vi "Roller Button Read.vi"(7 "Driver Button Cluster":T1, 9 "D-Pad":T2, 10 "Button Cluster":T1, 11 "Axes":T3) -> ()   [LabVIEW 2015]
uses:
  Real-Life Controls/Axes Cluster.ctl
  Real-Life Controls/D-Pad.ctl
  Real-Life Controls/Button Cluster.ctl
  Roller Modes.ctl
  Common Code/Auto Roller Commands.ctl
  Common Code/Roller Mode Enum.ctl
  Really Real Manual Align.ctl
  Common Code/Elevator State.ctl
  Common Code/Change Detect.vi
  Common Code/Change Detect Boolean.vi
  Robot Global Data.vi
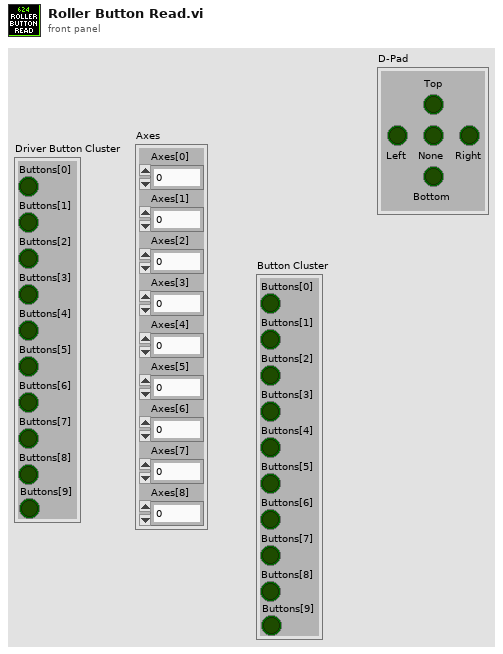
[diagram p1: front panel]
types:
  T1 = typedef "Button Cluster.ctl" = cluster{"Buttons[0]":bool, "Buttons[1]":bool, "Buttons[2]":bool, "Buttons[3]":bool, "Buttons[4]":bool, "Buttons[5]":bool, "Buttons[6]":bool, "Buttons[7]":bool, "Buttons[8]":bool, "Buttons[9]":bool}
  T2 = typedef "D-Pad.ctl" = cluster{"Top":bool, "Bottom":bool, "None":bool, "Right":bool, "Left":bool}
  T3 = typedef "Axes Cluster.ctl" = cluster{"Axes[0]":dbl, "Axes[1]":dbl, "Axes[2]":dbl, "Axes[3]":dbl, "Axes[4]":dbl, "Axes[5]":dbl, "Axes[6]":dbl, "Axes[7]":dbl, "Axes[8]":dbl}
  T4 = typedef "Elevator State.ctl" = enum16{"Idle", "Goto Load Position", "Wait for Load", "Load Drop", "Load Lift", "Drop Stack", "Goto Eject Position", "Eject ", "Raise Trashcan", "Open Stabilizer", "Untip Drop", "Untip Wait", "Untip Lift", "Abort Load", "HP Load Wait", "HP Load Drop", "HP Load Lift", "HP Load Abort", "Close Stabilizer", "HP Load Unfinish", "HP Load Score", "HP Load Finish", "HP Goto Finish Down", "HP Goto Finish Up", "Full"}
  T5 = typedef "Really Real Manual Align.ctl" = enum16{"In", "Left", "Right", "Out", "Idle", "HP Load", "Speeds"}
  T6 = typedef "Auto Roller Commands.ctl" = enum16{"Drag Tote", "Grab Tote", "Idle", "Eject Tote", "Untip Can", "Grab Can"}
  T7 = typedef "Roller Modes.ctl" = cluster{"Auto Roller Command":T6, "Roller Mode":T8, "Override Intake Speed":dbl}
  T8 = typedef "Roller Mode Enum.ctl" = enum16{"Manual", "Safe", "Auto"}
  T9 = typedef "Elevator Status.ctl" = cluster{"Height":dbl, "Enc Value":dbl, "Limit Override":bool, "Mode":T10, "High IR":bool, "Motor Out":dbl, "Ping Detect":bool, "Auto Elevator Indicators":T11, "Master Current":dbl, "Slave Current":dbl, "High Current":bool, "Current Tripped":bool, "Top Limit":bool, "Bottom Limit":bool, "Eject Piston":bool, "Stabilizer":bool, "Finger":bool, "Finger Height":dbl, "Finger Raw":dbl, "Finger at Bottom":bool}
  T10 = typedef "Elevator Mode.ctl" = enum16{"Manual", "Safe", "Auto"}
  T11 = typedef "Auto Elevator Indicators.ctl" = cluster{"Target Out":dbl, "Storing Trashcan?":bool, "State":T4, "In Range":bool, "Store Can Command":bool, "HP Load":bool}
  T12 = typedef "Dashboard Control Data.ctl" = cluster{"Cam Exposure":dbl, "Go to angle":dbl, "Steer PID Gains":cluster{"proportional gain (Kc)":dbl, "integral time (Ti, min)":dbl, "derivative time (Td, min)":dbl}, "Steer PID output Range":cluster{"output high":dbl, "output low":dbl}, "Pressure m \nValue":dbl, "Pressure b \nValue":dbl, "Roller Command Cluster ":T13, "Elevator":T14, "Encoder Control":T16, "Auton Settings":cluster{"Drive Dist Window Size":dbl}, "Drivetrain Settings":T17, "Lance":T18}
  T13 = typedef "Roller Control.ctl" = cluster{"Intake Speed":dbl, "Turn In Speed":dbl, "Unload Speed":dbl, "Turn Out Speed":dbl, "Ping Align Tolerance":dbl, "Tote Range Threshold":dbl, "Right Pot 0":dbl, "Pot Threshold":dbl, "Left Pot 0":dbl, "Right Pot Scale":dbl, "Left Pot Scale":dbl, "Min Elevator Height":dbl, "Eject Time":dbl, "Eject US Threshold":dbl, "Anti-Twitch Time":u32, "Ping Caring Threshold":dbl, "Pot Diff Threshold":dbl, "Pinch Sustain":u32, "Absorb Give Up Threshold":dbl, "Untip In Threshold":dbl, "Untip Grab Range":dbl, "Ultrasonic Hold Time":u32, "Landscape Absorb Time":u32, "Pot Use Wait Time":u32, "Can Turn Stop Range":dbl, "HP Load Speed":dbl, "Stick Multiplier":dbl, "Coop Eject Speed":dbl}
  T14 = typedef "Elevator DB Control.ctl" = cluster{"PID Output Range":cluster{"output high":dbl, "output low":dbl}, "PID gains":cluster{"proportional gain (Kc)":dbl, "integral time (Ti, min)":dbl, "derivative time (Td, min)":dbl}, "Height Tolerance":sgl, " Encoder Constant":dbl, "Eject Time":sgl, "Zeroing Speed":sgl, "Presets":T15, "Ping Detect Threshold":sgl, "Trashcan Detect Threshold":sgl, "Zero Filter Time":dbl, "Stabilizer Open Time":dbl, "Zero Creep Speed":dbl, "Max Current":dbl, "Current Trip Time":dbl, "Abort Pitch":dbl, "Finger m":dbl, "Finger b":dbl, "Finger max ":dbl, "Finger Stabilizer":dbl, "Finger Store":dbl, "Finger Stop Store":dbl, "Stabilizer Close Time":dbl, "Finger min":dbl, "Unstick gain":dbl, "Full Detect Max":dbl}
  T15 = typedef "Elevator Presets.ctl" = cluster{"Pickup 2 w/ Tote":sgl, "Pickup 2 w/ Trashcan":sgl, "Pickup 3 w/ Tote":sgl, "Pickup 3 w/ Trashcan":sgl, "Bottom":sgl, "Pickup 1 w/ Tote":sgl, "Pickup Trashcan":sgl, "Pickup 1 w/ Trashcan":sgl, "Eject":sgl, "Hold Low":sgl, "Step add height":sgl, "Untip Lift":dbl, "Drop Stack":dbl, "HP Load Hold":dbl, "HP Load Drop":dbl, "HP Load Hold Can":dbl, "Store can max":dbl, "HP Drag Score":dbl, "HP Drag Finish":dbl, "Finger trashcan avoid":dbl, "Full":dbl}
  T16 = typedef "Encoder Control.ctl" = cluster{"Left Tick Constant":dbl, "Right Tick Constant":dbl, "Center Tick Constant":dbl, "Reset?":bool, "Y Dist":cluster{"PID gains":cluster{"proportional gain (Kc)":dbl, "integral time (Ti, min)":dbl, "derivative time (Td, min)":dbl}}, "X Dist":cluster{"PID gains":cluster{"proportional gain (Kc)":dbl, "integral time (Ti, min)":dbl, "derivative time (Td, min)":dbl}}, "Y Stop Thresh":dbl, "Y Stop Speed":dbl, "X Stop Thresh":dbl, "X Stop Speed":dbl}
  T17 = typedef "Drivetrain Settings.ctl" = cluster{"Gyro Tolerance":sgl, "Strafe Correct max steer":sgl, "Strafe Timer Wait":sgl, "Throttle Ramp (ms)":sgl, "Strafe Ramp (ms)":sgl, "Angular rate compensation":bool, "Throttle to Rate Scale":sgl, "Rate compensation gain":sgl, "Creep Steer":sgl, "Creep Throttle":sgl}
  T18 = typedef "Pike DB Controls.ctl" = cluster{"Down Speed":dbl, "Up Speed":dbl, "Max Down Time":dbl, "Max Up Time":dbl, "Current Limit":dbl}
  T19 = typedef "Roller Manual Bools.ctl" = cluster{"Manual Claw":bool, "Manual Align":T5, "Left Speed":dbl, "Right Speed":dbl}
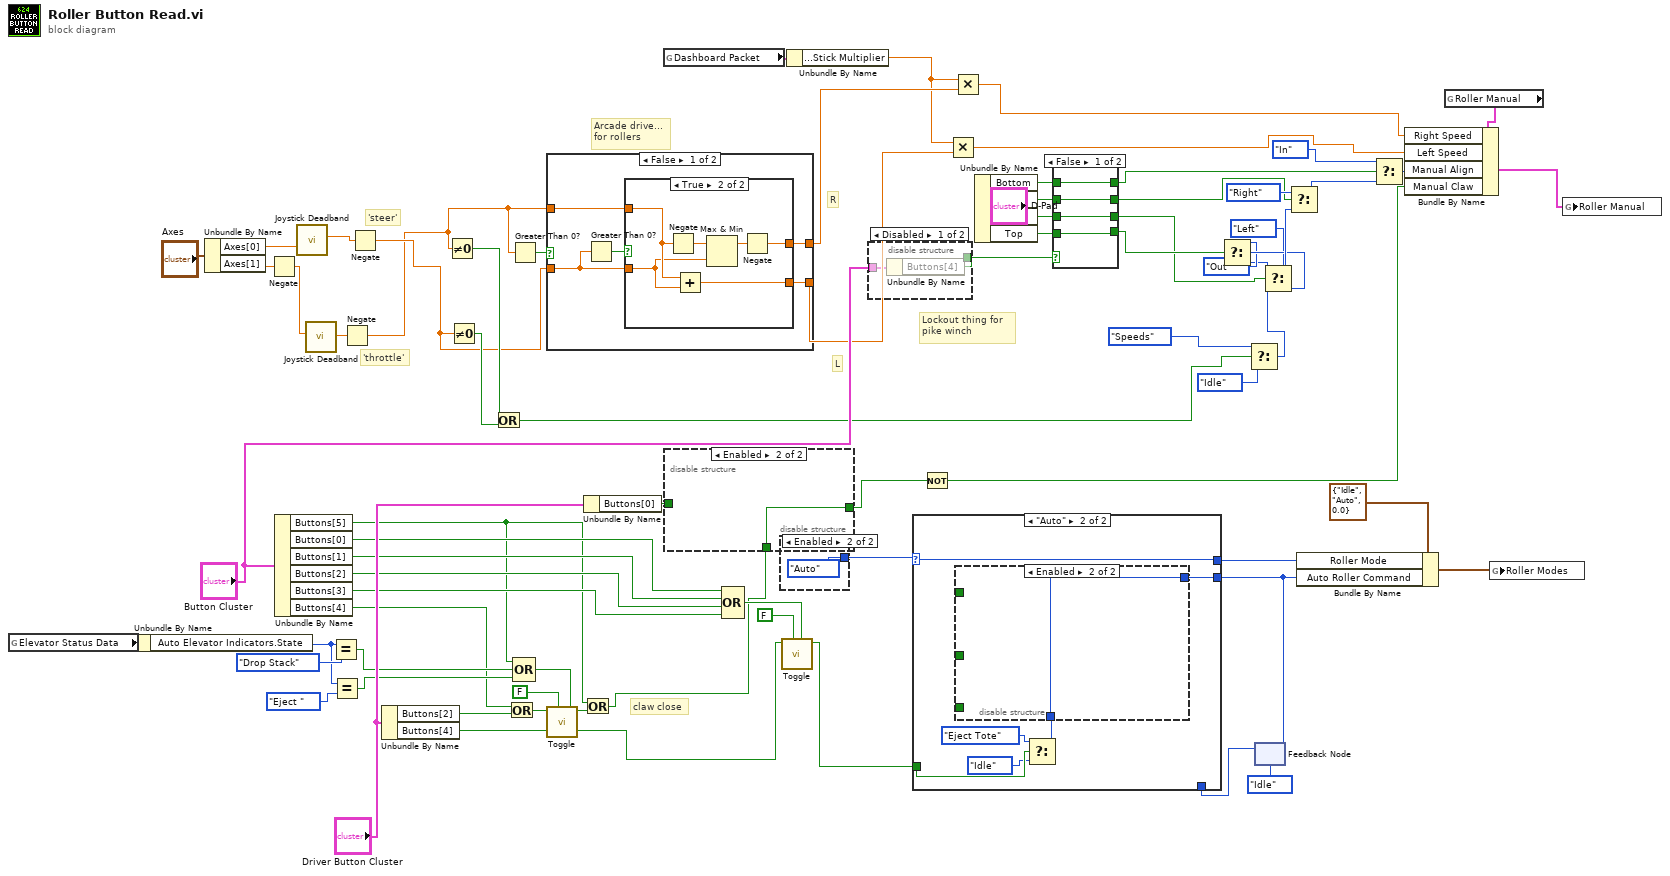
[diagram p0: block diagram]
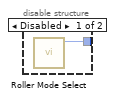
[diagram p2: hidden frame]
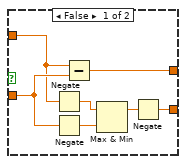
[diagram p5: hidden frame]
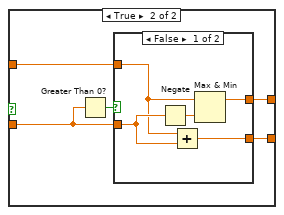
[diagram p6: hidden frame]
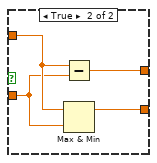
[diagram p7: hidden frame]
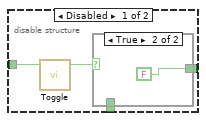
[diagram p8: hidden frame]
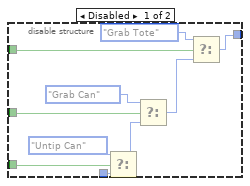
[diagram p11: hidden frame]
diagram:
  # "claw close"
  # "Lockout thing for\npike winch"
  # "'steer'"
  # "'throttle'"
  # "L"
  # "R"
  # "Arcade drive...\nfor rollers"
  n1 = global read "Robot Global Data.vi" "Elevator Status Data"() -> (w11:T9)
  n2 = Unbundle By Name(w11) -> ("Auto Elevator Indicators.State"=w6:T4)
  n3 = Unbundle By Name("Axes") -> ("Axes[0]"=w48:dbl, "Axes[1]"=w49:dbl)
  n4 = Negate(x=w49) -> (-x=w47:dbl)
  n5 = Unbundle By Name("Button Cluster") -> ("Buttons[5]"=w4:bool, "Buttons[0]"=w22:bool, "Buttons[1]"=w21:bool, "Buttons[2]"=w20:bool, "Buttons[3]"=w19:bool, "Buttons[4]"=w2:bool)
  n6 = call "Joystick Deadband.vi"("In"=w48) -> ("Out"=w41:dbl)  [unwired: 10 in]
  n7 = call "Joystick Deadband.vi"("In"=w47) -> ("Out"=w38:dbl)  [unwired: 10 in]
  n8 = Equal?(x=w6, y=Elevator_State."Drop Stack") -> (x = y?=w9:bool)
  n9 = Equal?(x=w6, y=Elevator_State."Eject ") -> (x = y?=w5:bool)
  n10 = Negate(x=w38) -> (-x=w39:dbl)
  n11 = Negate(x=w41) -> (-x=w40:dbl)
  n12 = Unbundle By Name("Driver Button Cluster") -> ("Buttons[2]"=w3:bool, "Buttons[4]"=w16:bool)
  n13 = Not Equal To 0?(x=w39) -> (x != 0?=w45:bool)
  n14 = Not Equal To 0?(x=w40) -> (x != 0?=w46:bool)
  n15 = Or(x=w45, y=w46) -> (x .or. y?=w43:bool)
  n16 = Or(x=w2, y=w3) -> (x .or. y?=w1:bool)
  n17 = Greater Than 0?(x=w39) -> (x > 0?=w44:bool)
  n18 = Compound Arithmetic op=OR(w4, w9, w5) -> (w8:bool)
  n19 = case shown="False" w44 {
    tunnel: w40 -> [w79 w97]
    tunnel: w39 -> [w78 w96]
    tunnel: [w77 w95] -> w24
    tunnel: [w76 w94] -> w27
    frame False {
      n20 = Greater Than 0?(x=w79) -> (x > 0?=w80:bool)
      n21 = case shown="True" w80 {
        tunnel: w79 -> [w87 w89]
        tunnel: w78 -> [w85 w90]
        tunnel: [w81 w91] -> w77
        tunnel: [w82 w88] -> w76
        frame False {
          n22 = Negate(x=w85) -> (-x=w86:dbl)
          n23 = Negate(x=w87) -> (-x=w84:dbl)
          n24 = Subtract(x=w85, y=w87) -> (x-y=w81:dbl)
          n25 = Max & Min(x=w86, y=w84) -> (max(x,y)=w83:dbl)  [unwired: 1 out]
          n26 = Negate(x=w83) -> (-x=w82:dbl)
        }
        frame True {
          n27 = Negate(x=w90) -> (-x=w93:dbl)
          n28 = Add(x=w90, y=w89) -> (x+y=w88:dbl)
          n29 = Max & Min(x=w93, y=w89) -> (max(x,y)=w92:dbl)  [unwired: 1 out]
          n30 = Negate(x=w92) -> (-x=w91:dbl)
        }
      }
    }
    frame True {
      n31 = Greater Than 0?(x=w97) -> (x > 0?=w98:bool)
      n32 = case shown="False" w98 {
        tunnel: w97 -> [w103 w105]
        tunnel: w96 -> [w100 w106]
        tunnel: [w101 w104] -> w95
        tunnel: [w99 w107] -> w94
        frame False {
          n33 = Negate(x=w103) -> (-x=w102:dbl)
          n34 = Add(x=w100, y=w103) -> (x+y=w99:dbl)
          n35 = Max & Min(x=w100, y=w102) -> (max(x,y)=w101:dbl)  [unwired: 1 out]
        }
        frame True {
          n36 = Subtract(x=w106, y=w105) -> (x-y=w104:dbl)
          n37 = Max & Min(x=w106, y=w105) -> (max(x,y)=w107:dbl)  [unwired: 1 out]
        }
      }
    }
  }
  n38 = call "Toggle.vi"("Reinit?"=w8, "Initial Value"=FALSE, "In"=w1) -> ("Toggled"=w14:bool)  [unwired: 8 in]
  n39 = Or(x=w4, y=w14) -> (x .or. y?=w12:bool)
  n40 = Unbundle By Name("Driver Button Cluster") -> ("Buttons[0]"=w61:bool)
  n41 = global read "Robot Global Data.vi" "Dashboard Packet"() -> (w28:T12)
  n42 = disable-structure shown="Enabled" {
    disable-tunnel: [w110 w114] -> w65
    disable-tunnel: w61 -> [w109 _]
    disable-tunnel: w12 -> [w108 w114]
    frame Disabled {
      n43 = call "Toggle.vi"("In"=w109) -> ("Toggled"=w111:bool)  [unwired: 10 in]
      n44 = case shown="True" w111 {
        tunnel: [w112 FALSE] -> w110
        tunnel: w108 -> [w112 _]
        frame False {
        }
        frame True {
        }
      }
    }
    frame Enabled {
    }
  }
  n45 = Compound Arithmetic op=OR(w22, w21, w20, w19) -> (w18:bool)
  n46 = disable-structure shown="Enabled" {
    disable-tunnel: [w115 Roller_Mode_Enum."Auto" ("Mode")] -> w69
    frame Disabled {
      n47 = call "Roller Mode Select.vi"() -> ("Mode"=w115:T8)  [unwired: 11 in]
    }
    frame Enabled {
    }
  }
  n48 = call "Toggle.vi"("Reinit?"=w18, "Initial Value"=FALSE, "In"=w16) -> ("Toggled"=w15:bool)  [unwired: 8 in]
  n49 = Unbundle By Name(w28) -> ("Roller Command Cluster.Stick Multiplier"=w23:dbl)
  n50 = disable-structure shown="Disabled" {
    disable-tunnel: "Button Cluster" -> [w118 _]
    disable-tunnel: [w117 _] -> w31
    frame Disabled {
      n51 = Unbundle By Name(w118) -> ("Buttons[4]"=w117:bool)
    }
    frame Enabled {
    }
  }
  n52 = Not(x=w65) -> (.not. x?=w64:bool)
  n53 = Multiply(x=w23, y=w27) -> (x*y=w26:dbl)
  n54 = Multiply(x=w23, y=w24) -> (x*y=w25:dbl)
  n55 = Unbundle By Name("D-Pad") -> ("Bottom"=w36:bool, "Right"=w35:bool, "Left"=w34:bool, "Top"=w33:bool)
  n56 = case shown="False" w31 {
    tunnel: [w119 _] -> w30
    tunnel: w33 -> [w119 _]
    tunnel: w34 -> [w121 _]
    tunnel: [w121 _] -> w29
    tunnel: w35 -> [w120 _]
    tunnel: [w120 _] -> w32
    tunnel: w36 -> [w122 _]
    tunnel: [w122 _] -> w37
    frame False {
    }
    frame True {
    }
  }
  n57 = Select(t=Really_Real_Manual_Align."Speeds", s=w43, f=Really_Real_Manual_Align."Idle" ("Manual Align")) -> (s? t:f=w50:T5)
  n58 = Select(t=Really_Real_Manual_Align."Out" ("Manual Align"), s=w30, f=w50) -> (s? t:f=w57:T5)
  n59 = feedback #1(Auto_Roller_Commands."Idle" ("Auto Roller State")) -> (w70:T6)
  n60 = case shown="\"Auto\"" w69 {
    selector: w69 -> [w123 w129]
    tunnel: [w124 w130] -> w72
    tunnel: w70 -> [w124 _]
    tunnel: [w123 w129] -> w71
    tunnel: w15 -> [_ w128]
    frame "Manual", Default {
    }
    frame "Auto" {
      n61 = Select(t=Auto_Roller_Commands."Eject Tote" ("Auto Roller State"), s=w128, f=Auto_Roller_Commands."Idle" ("Auto Roller State")) -> (s? t:f=w125:T6)
      n62 = disable-structure shown="Enabled" {
        disable-tunnel: [w140 w141] -> w130
        disable-tunnel: _ -> [w139 _]
        disable-tunnel: _ -> [w138 _]
        disable-tunnel: w125 -> [w133 w141]
        disable-tunnel: _ -> [w132 _]
        frame Disabled {
          n63 = Select(t=Auto_Roller_Commands."Untip Can", s=w139, f=w133) -> (s? t:f=w137:T6)
          n64 = Select(t=Auto_Roller_Commands."Grab Can", s=w138, f=w137) -> (s? t:f=w131:T6)
          n65 = Select(t=Auto_Roller_Commands."Grab Tote" ("Auto Roller State"), s=w132, f=w131) -> (s? t:f=w140:T6)
        }
        frame Enabled {
        }
      }
    }
  }
  n66 = feedback-in #1(w72) -> ()
  n67 = Select(t=Really_Real_Manual_Align."Left" ("Manual Align"), s=w29, f=w57) -> (s? t:f=w58:T5)
  n68 = Select(t=Really_Real_Manual_Align."Right" ("Manual Align"), s=w32, f=w58) -> (s? t:f=w59:T5)
  n69 = Bundle By Name(cluster=T7 {"Auto Roller Command"=enum."Idle", "Roller Mode"=enum."Auto", "Override Intake Speed"=0.0} ("Roller Modes"), "Roller Mode"=w71, "Auto Roller Command"=w72) -> (w67:T7)
  n70 = Select(t=Really_Real_Manual_Align."In" ("Manual Align"), s=w37, f=w59) -> (s? t:f=w52:T5)
  n71 = global read "Robot Global Data.vi" "Roller Manual"() -> (w73:T19)
  n72 = Bundle By Name(cluster=w73, "Right Speed"=w25, "Left Speed"=w26, "Manual Align"=w52, "Manual Claw"=w64) -> (w74:T19)
  n73 = global write "Robot Global Data.vi" "Roller Modes"(w67) -> ()
  n74 = global write "Robot Global Data.vi" "Roller Manual"(w74) -> ()
